vi "Initialize Instrument.vi"(8 "error in (no error)":errorcluster, 10 "Instr Resource Str":string, 11 "Simulated Scope.lvclass in":refnum<class "Simulated Scope.lvclass">) -> (0 "error out":errorcluster, 3 "Simulated Scope.lvclass out":refnum<class "Simulated Scope.lvclass">)   [LabVIEW 2010, in "Simulated Scope.lvclass"]
doc: "Initialize VI for the Simulated Scope Class"
uses:
  Simulated Scope.lvclass
  Simulated Scope Operation.ctl
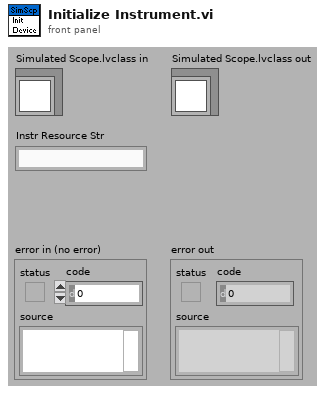
[diagram p1: front panel]
types:
  T1 = typedef "Simulated Scope.lvclass/Simulated Scope Operation.ctl" = enum16{"Read", "Clear"}
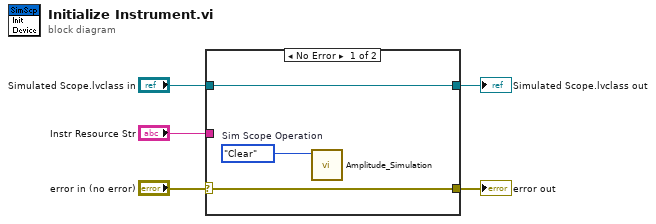
[diagram p0: block diagram]
diagram:
  n1 = case shown="No Error" "error in (no error)" {
    selector: "error in (no error)" -> [w7 w10]
    tunnel: [w7 w10] -> w4
    tunnel: "Simulated Scope.lvclass in" -> [w8 w9]
    tunnel: [w8 w9] -> w5
    tunnel: "Instr Resource Str" -> [_ _]
    frame No Error {
      w6 = Simulated_Scope_Operation."Clear"  # Sim Scope Operation
      n2 = call "Amplitude_Simulation.vi"("Sim Scope Operation"=w6) -> ()  [unwired: 11 out]
    }
    frame Error {
    }
  }
  "error out" <- w4
  "Simulated Scope.lvclass out" <- w5
